vi "maximo.vi"(8 "error in (no error)":errorcluster, 10 "maximo":dbl, 11 "Status Actor in":refnum<class "Status Actor.lvclass">) -> (0 "error out":errorcluster, 3 "Status Actor out":refnum<class "Status Actor.lvclass">)   [LabVIEW 2019, in "Status Actor.lvlib" / "Status Actor.lvclass"]
uses:
  Status Actor.lvclass
  Status Actor.lvclass/Status Actor.ctl
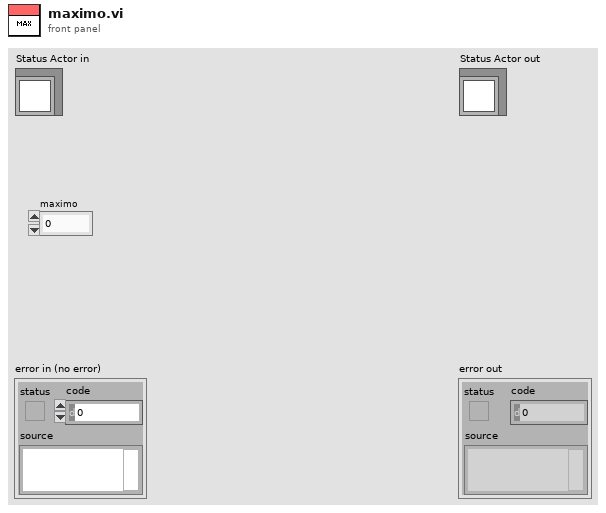
[diagram p1: front panel]
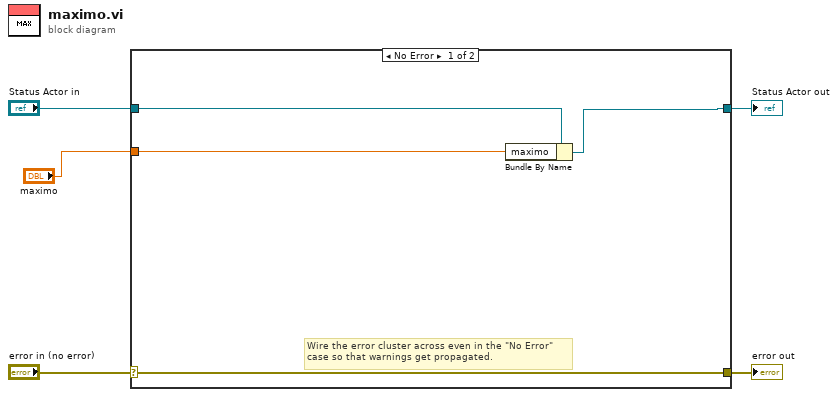
[diagram p0: block diagram]
diagram:
  n1 = case shown="No Error" "error in (no error)" {
    selector: "error in (no error)" -> [w9 w11]
    tunnel: [w9 w11] -> w4
    tunnel: [w6 w10] -> w2
    tunnel: "Status Actor in" -> [w7 w10]
    tunnel: "maximo" -> [w8 _]
    frame No Error {
      # "Wire the error cluster across even in the \"No Error\"\ncase so that warnings get propagated."
      n2 = Bundle By Name(cluster=w7, "maximo"=w8) -> (w6:refnum<class "Status Actor.lvclass">)
    }
    frame Error {
    }
  }
  "error out" <- w4
  "Status Actor out" <- w2
